vi "Miniquads.destructor.vi"(0 "i ref in":refnum<vi>, 5 "error in (no error)":errorcluster) -> (19 "error out":errorcluster)   [LabVIEW 2014, in "Miniquads.lvlib"]
doc: "This is the destructor of a class.\n\nLicense Agreement for this software:\n\nCopyright (C) 2011 Christopher Borgmann\nMax-Planck-Institut für Kernphysik\nSaupfercheckweg 1\n69117 Heidelberg\nGermany\n\nThis program is free software: you can redistribute it and/or modify it under the terms of the GNU General Public License as published by the Free Software Foundation, either version 3 of the License, or (at your option) any later version.\n\nThis program is distributed in the hope that it will be useful, but WITHOUT ANY WARRANTY; without even the implied warranty of MERCHANTABILITY or FITNESS FOR A PARTICULAR PURPOSE. See the GNU General Public License for more details.\n\nYou should have received a copy of the GNU General Public License along with this program. If not, see <http://www.gnu.org/licenses/>.\n\nFor all questions and ideas contact: christopher.borgmann@cern.ch."
uses:
  Miniquads.lvlib
  CSCore/CSApplicationBaseClasses/DeviceBase/DeviceBase.lvlib
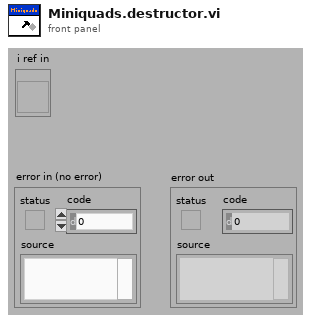
[diagram p1: front panel]
types:
  T1 = enum16{"SetAttribute", "GetAttribute", "CreateAttribute", "DestroyAttribute", "DestroyAllAtributes"}
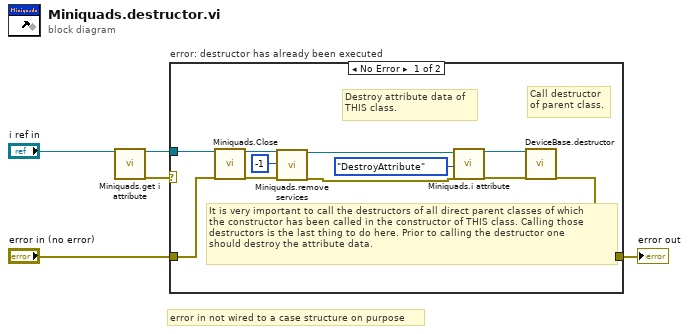
[diagram p0: block diagram]
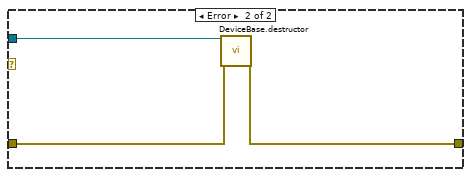
[diagram p2: hidden frame]
diagram:
  # "error in not wired to a case structure on purpose"
  n1 = call "Miniquads.get i attribute.vi"("i ref in"="i ref in") -> ("i ref out"=w1:refnum<vi>, "error out"=w2:errorcluster)  [unwired: 16 in, 1 out]
  n2 = case "error: destructor has already been executed" shown="No Error" w2 {
    tunnel: [w13 w17] -> w5
    tunnel: "error in (no error)" -> [w11 w18]
    tunnel: w1 -> [w12 w19]
    frame No Error {
      # "It is very important to call the destructors of all direct parent classes of which\nthe constructor has been called in the constructor of THIS class. Calling those\ndestructors is the last thing to do here. Prior to calling the destructor one \nshould destroy the attribute data."
      # "Destroy attribute data of \nTHIS class."
      # "Call destructor\nof parent class."
      n3 = call "Miniquads.Close.vi"("i ref in"=w12, "error in (no error)"=w11) -> ("i ref out"=w10:refnum<vi>, "error out"=w9:errorcluster)  [unwired: 15 in, 1 out]
      n4 = call "Miniquads.remove services.vi"("i ref in"=w10, "ms timeout (10000)"=-1, "error in (no error)"=w9) -> ("i ref out"=w8:refnum<vi>, "error out"=w7:errorcluster)  [unwired: 14 in, 1 out]
      n5 = call "Miniquads.i attribute.vi"("VI Refnum"=w8, "Action"=T1."DestroyAttribute", "error in (no error)"=w7) -> ("VI Refnum out"=w15:refnum<vi>, "error out"=w14:errorcluster)  [unwired: 14 in, 1 out]
      n6 = call "DeviceBase.destructor.vi"("i ref in"=w15, "error in (no error)"=w14) -> ("error out"=w13:errorcluster)  [unwired: 17 in]
    }
    frame Error {
      n7 = call "DeviceBase.destructor.vi"("i ref in"=w19, "error in (no error)"=w18) -> ("error out"=w17:errorcluster)  [unwired: 17 in]
    }
  }
  "error out" <- w5
